vi "CU_findBestNu.vi"(2 "Accuracy Graph":cluster{dbl[], dbl[]}[](graph)) -> (6 "Max Average Accuracy":dbl, 7 "Best Value":dbl, 10 "Average Accuracy":cluster{dbl[], dbl[]})   [LabVIEW 2016, in "Classifier.lvlib"]
uses:
  Classifier.lvlib
panel:
  # "This VI is a part of BCI Design library, http://www.ru-bci.org \nCopyright © 2020, Sotnikov Peter, All rights reserved. License: GNU GPLv3"
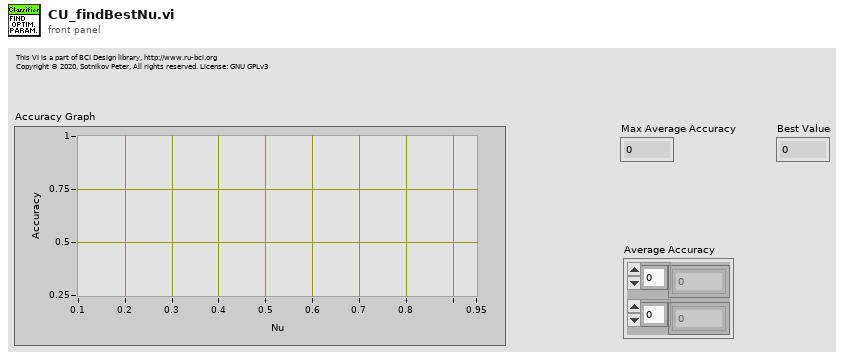
[diagram p1: front panel]
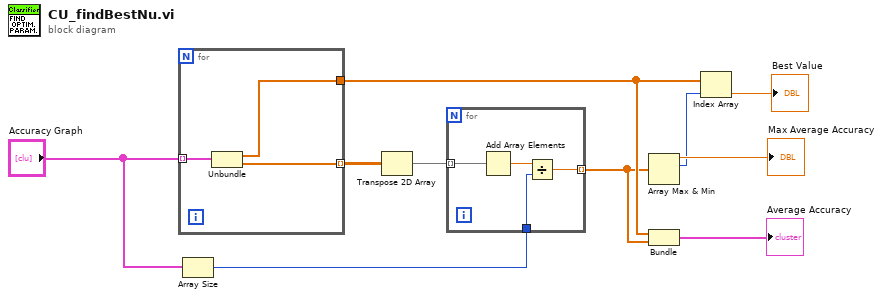
[diagram p0: block diagram]
diagram:
  n1 = for {
    tunnel: "Accuracy Graph" -> [w13] mode=indexing
    tunnel: [w12] -> w10 mode=indexing
    tunnel: [w11] -> w3
    n2 = Unbundle(w13) -> (w11:dbl[], w12:dbl[])
  }
  n3 = Array Size(array="Accuracy Graph") -> (size(s)=w7:i32)
  n4 = Transpose 2D Array(2D array=w10) -> (transposed array=w8:dbl[][])
  n5 = for {
    tunnel: w8 -> [w17] mode=indexing
    tunnel: w7 -> [w15]
    tunnel: [w14] -> w2 mode=indexing
    n6 = Add Array Elements(numeric array=w17) -> (sum=w16:dbl)
    n7 = Divide(x=w16, y=w15) -> (x/y=w14:dbl)
  }
  n8 = Array Max & Min(array=w2) -> (max value=→"Max Average Accuracy":dbl, max index (indices)=w5:i32)  [unwired: 2 out]
  n9 = Bundle(w3, w2) -> (→"Average Accuracy":cluster{dbl[], dbl[]})  [unwired: 1 in]
  n10 = Index Array(array=w3, index=w5) -> (element=→"Best Value":dbl)
